vi "Pre-Build Action.vi"(6 "Top Level/Always Included VIs":path[](array[path]) caption="VIs Niveau principal/Toujours inclus", 7 "Main Destination Path":path caption="Chemin de destination principal", 9 "Target Name":string caption="Nom de la cible", 10 "Build Specification Name":string caption="Nom de la spécification de construction", 11 "Project Path":path caption="Chemin du projet") -> (0 "error out":errorcluster caption="sortie d'erreur")   [LabVIEW 2020]
panel:
  in  "error in (no error)":errorcluster caption="entrée d'erreur (pas d'erreur)"
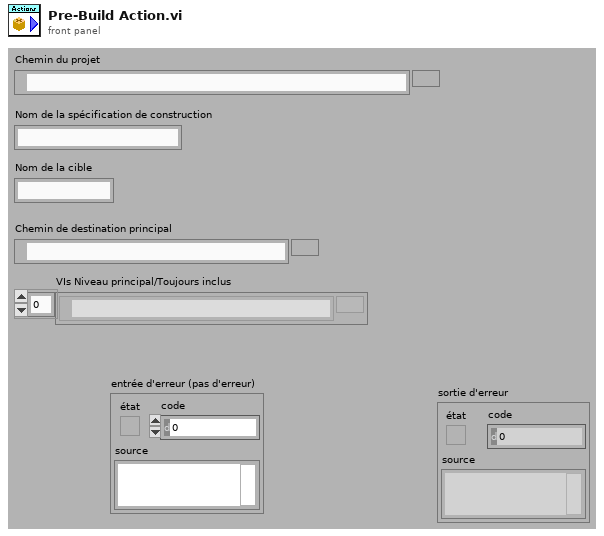
[diagram p1: front panel]
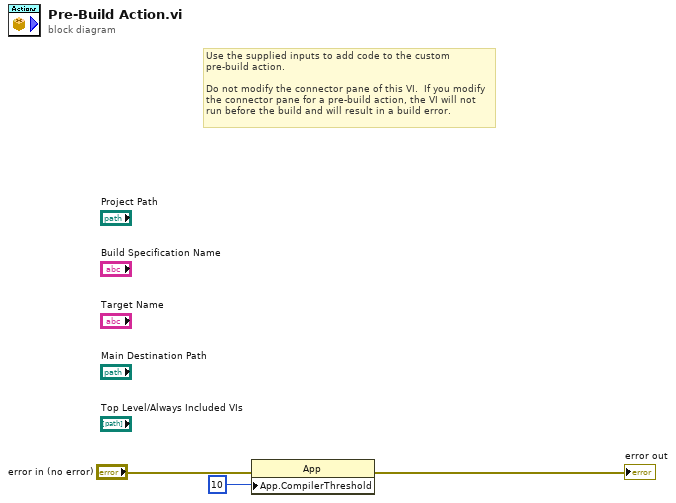
[diagram p0: block diagram]
diagram:
  # "Use the supplied inputs to add code to the custom pre-build action.\n\nDo not modify the connector pane of this VI.  If you modify the connector pane for a pre-build action, the VI will not run before the build and will result in a build error."
  n1 = property class="App"(error in="error in (no error)", "App.CompilerThreshold"=u32 10 ("Application:Seuil du compilateur")) -> (error out=→"error out":errorcluster)  [unwired: 1 in, 1 out]
